vi "testGetSetting.vi"(8 "error in (no error)":errorcluster) -> (0 "error out":errorcluster)   [LabVIEW 2016]
doc: "Test to read the configuration file based on the Parameter."
uses:
  <vilib>/addons/_JKI Toolkits/Caraya/classes/Assert/Assert.lvclass
  <vilib>/addons/_JKI Toolkits/Caraya/classes/Test/Test.lvclass
  MatOper/MatOper.lvclass
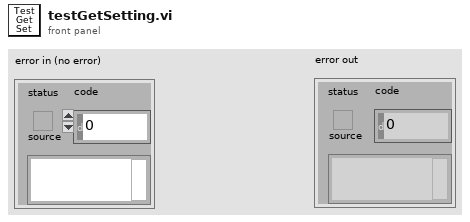
[diagram p1: front panel]
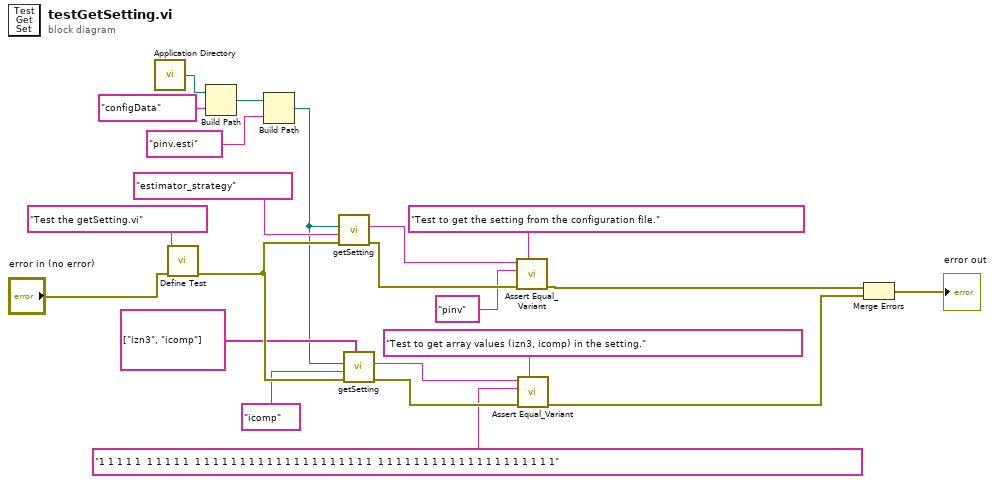
[diagram p0: block diagram]
diagram:
  n1 = call <vilib>:"Application Directory.vi"() -> ("Application Directory"=w5:path)
  n2 = call <vilib>:"Define Test.vi"("error in (no error)"="error in (no error)", "Label (VI Title)"="Test the getSetting.vi") -> ("error out"=w15:errorcluster)  [unwired: 9 in]
  n3 = Build Path(base path=w5, name or relative path="configData") -> (appended path=w3:path)
  n4 = Build Path(base path=w3, name or relative path="pinv.esti") -> (appended path=w1:path)
  n5 = call "getSetting.vi"("error in (no error)"=w15, "Parameter"="estimator_strategy", "Path"=w1) -> ("error out"=w19:errorcluster, "Value"=w17:string)  [unwired: 6 in, 1 out]
  n6 = call "getSetting.vi"("Array Parameter List"=string[] ["izn3", "icomp"], "error in (no error)"=w15, "Parameter"="icomp", "Path"=w1) -> ("error out"=w11:errorcluster, "Value"=w12:string)  [unwired: 5 in, 1 out]
  n7 = call <vilib>:"Assert Equal_Variant.vi"("Label"="Test to get the setting from the configuration file.", "error in (no error)"=w19, "Y"="pinv" ("Value"), "X"=w17) -> ("error out"=w8:errorcluster)  [unwired: 7 in]
  n8 = call <vilib>:"Assert Equal_Variant.vi"("Label"="Test to get array values (izn3, icomp) in the setting.", "error in (no error)"=w11, "Y"="1 1 1 1 1  1 1 1 1 1  1 1 1 1 1 1 1 1 1 1 1 1 1 1 1 1 1 1 1 1  1 1 1 1 1 1 1 1 1 1 1 1 1 1 1 1 1 1 1 1", "X"=w12) -> ("error out"=w7:errorcluster)  [unwired: 7 in]
  n9 = Merge Errors(w8, w7) -> (→"error out":errorcluster)
